vi "SVI_SerialReceive.vi"(6 "End Char":string="\n", 7 "Wait time (ms)":u32=1000, 8 "error in (no error)":errorcluster, 11 "VISA Refnum in":refnum<visa-resource-name>) -> (0 "error out":errorcluster, 2 "read buffer":string, 3 "VISA resource name out":refnum<visa-resource-name>)   [LabVIEW 2014]
panel:
  out "Numeric Control":i32
  out "Array":u32[](array[numeric])
  out "x-y":u32
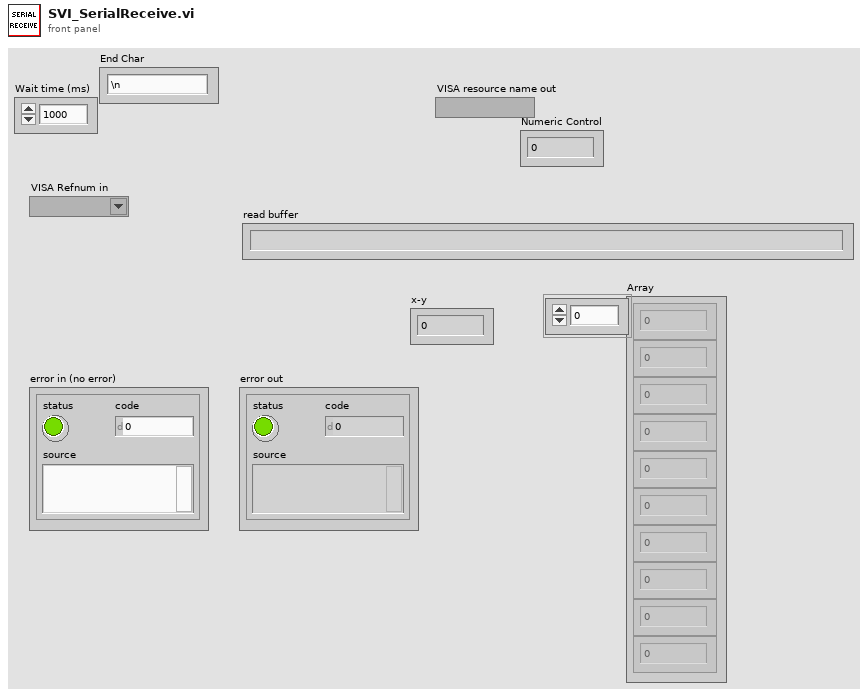
[diagram p1: front panel]
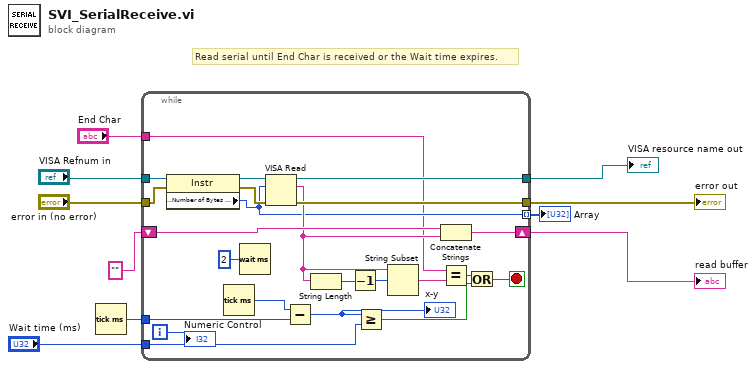
[diagram p0: block diagram]
diagram:
  # "Read serial until End Char is received or the Wait time expires."
  n1 = Tick Count (ms)() -> (millisecond timer value=w4:u32)
  n2 = while {
    tunnel: "VISA Refnum in" -> [w31]
    tunnel: [w29] -> w7
    shift-right: [w14] -> w5
    shift-left: "" -> [w27]
    tunnel: w4 -> [w22]
    tunnel: "error in (no error)" -> [w30]
    tunnel: [w28] -> w6
    tunnel: "Wait time (ms)" -> [w18]
    tunnel: [w15] -> w2 mode=indexing
    tunnel: "End Char" -> [w12]
    i -> [w11]
    stop <- w13 stop-if-true
    n3 = property class="Instr"(reference=w31, error in=w30) -> (reference out=w33:refnum<visa-resource-name>, error out=w32:errorcluster, "Serial Settings:Number of Bytes at Serial Port"=w15:u32)
    n4 = Tick Count (ms)() -> (millisecond timer value=w23:u32)
    n5 = Wait (ms)(milliseconds to wait=u32 2) -> ()  [unwired: 1 out]
    n6 = VISA Read(VISA resource name=w33, byte count=w15, error in (no error)=w32) -> (VISA resource name out=w29:refnum<visa-resource-name>, read buffer=w19:string, error out=w28:errorcluster)  [unwired: 1 out]
    n7 = Subtract(x=w23, y=w22) -> (x-y=w21:u32)
    "x-y" <- w21
    n8 = String Length(string=w19) -> (length=w25:i32)
    n9 = Decrement(x=w25) -> (x-1=w24:i32)
    n10 = Greater Or Equal?(x=w21, y=w18) -> (x >= y?=w17:bool)
    n11 = String Subset(string=w19, offset (0)=w24) -> (substring=w20:string)  [unwired: 1 in]
    n12 = Concatenate Strings(w27, w19) -> (w14:string)
    n13 = Equal?(x=w12, y=w20) -> (x = y?=w26:bool)
    n14 = Or(x=w26, y=w17) -> (x .or. y?=w13:bool)
    "Numeric Control" <- w11
  }
  "read buffer" <- w5
  "error out" <- w6
  "VISA resource name out" <- w7
  "Array" <- w2
